vi "Delete First Element.vi"(8 "error in (no error)":errorcluster, 11 "Cluster in":variant) -> (0 "error out":errorcluster, 1 "element":variant, 2 "Name":string, 3 "Cluster out":variant)   [LabVIEW 2020, in "Variant Data Manipulation.lvlib"]
uses:
  Variant Data Manipulation.lvlib
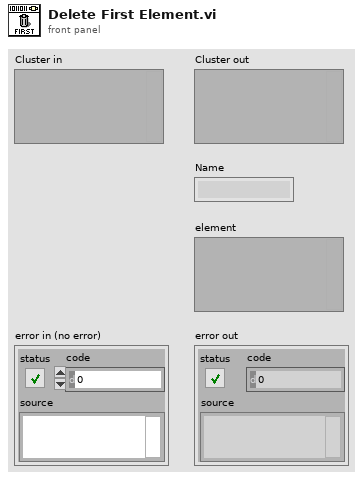
[diagram p1: front panel]
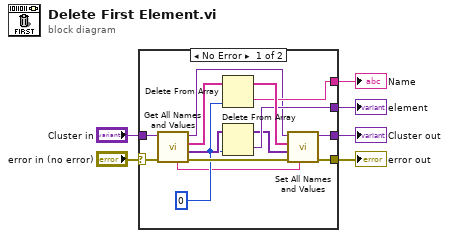
[diagram p0: block diagram]
diagram:
  n1 = case shown="No Error" "error in (no error)" {
    selector: "error in (no error)" -> [w20 w21]
    tunnel: [w18 w21] -> w5
    tunnel: [w17 w22] -> w4
    tunnel: "Cluster in" -> [w16 w22]
    tunnel: [w13 _] -> w2
    tunnel: [w12 _] -> w1
    frame No Error {
      w9 = 0 ("index")
      n2 = call "Get All Names and Values.vi"("error in"=w20, "Cluster in"=w16) -> ("error out"=w19:errorcluster, "Values"=w11:variant[], "Element Names"=w15:string[], "Cluster out"=w7:variant, "Cluster Name"=w8:string)  [unwired: 5 in]
      n3 = Delete From Array(array=w15, index=w9) -> (deleted portion=w13:string, array with subset deleted=w14:string[])  [unwired: 1 in]
      n4 = Delete From Array(array=w11, index=w9) -> (deleted portion=w12:variant, array with subset deleted=w10:variant[])  [unwired: 1 in]
      n5 = call "Set All Names and Values.vi"("Cluster Name"=w8, "error in"=w19, "values"=w10, "Element Names"=w14, "Cluster in"=w7) -> ("error out"=w18:errorcluster, "Cluster out"=w17:variant)  [unwired: 5 in]
    }
    frame Error {
    }
  }
  "Cluster out" <- w4
  "error out" <- w5
  "element" <- w1
  "Name" <- w2
